vi "Stop.vi"(8 "error in (no error)":errorcluster, 11 "FitterBase in":refnum<class "SaveWaveforms.lvclass">) -> (0 "error out":errorcluster, 3 "FitterBase out":refnum<class "SaveWaveforms.lvclass">)   [LabVIEW 2018, in "AnalysisPlugins.lvlib" / "SaveWaveforms.lvclass"]
uses:
  SaveWaveforms.lvclass
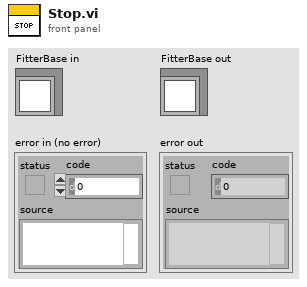
[diagram p1: front panel]
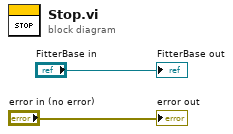
[diagram p0: block diagram]
diagram:
  "error out" <- "error in (no error)"
  "FitterBase out" <- "FitterBase in"
